vi "DSF.Engine.Transfer.Get id.vi"(11 "Transfer in":refnum<class "DSF.Engine.Transfer.lvclass">) -> (2 "id":T1, 3 "Transfer out":refnum<class "DSF.Engine.Transfer.lvclass">)   [LabVIEW 2017, in "DSF.Engine.lvlib" / "DSF.Engine.Transfer.lvclass"]
uses:
  DSF.Engine.Transfer.lvclass
  Typedefs/DSF.Engine.Typedefs.ID.ctl
  DSF.Engine.Transfer.lvclass/DSF.Engine.Transfer.ctl
  DSF.Engine.lvlib
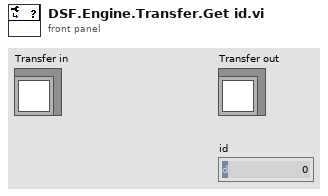
[diagram p1: front panel]
types:
  T1 = typedef "DSF.Engine.lvlib/DSF.Engine.Typedefs.ID.ctl" = i32
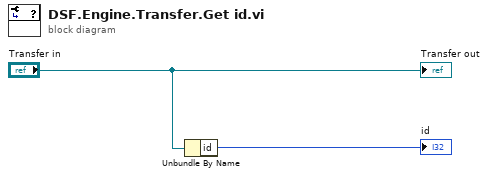
[diagram p0: block diagram]
diagram:
  n1 = Unbundle By Name("Transfer in") -> ("id"=→"id":T1)
  "Transfer out" <- "Transfer in"
